vi "Enum Strings.vi"(11 "Enum":variant) -> (2 "Selected item":string, 3 "Strings":string[](array[string]), 5 "# items in Enum":i16)   [LabVIEW 2011, in "LV JSON.lvlib"]
uses:
  LV JSON.lvlib
panel:
  out "selected item":u32
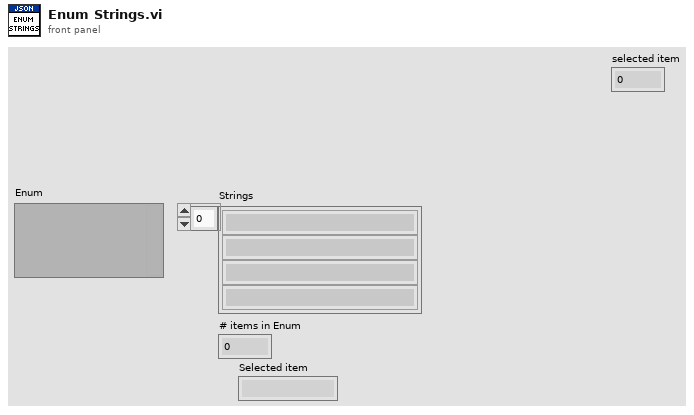
[diagram p1: front panel]
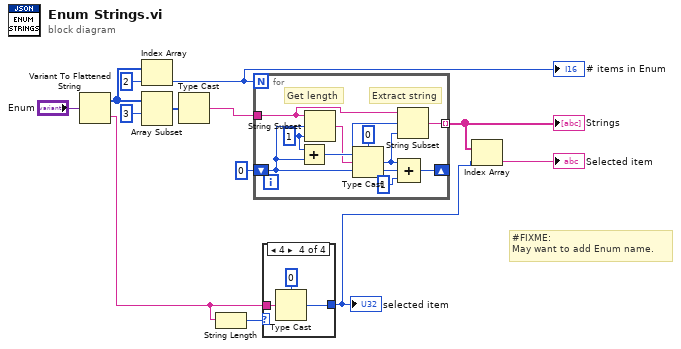
[diagram p0: block diagram]
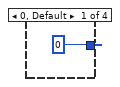
[diagram p2: hidden frame]
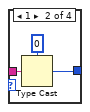
[diagram p3: hidden frame]
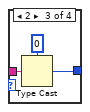
[diagram p4: hidden frame]
diagram:
  # "#FIXME:\nMay want to add Enum name."
  n1 = Variant To Flattened String(Variant="Enum") -> (data string=w4:string, 1:w11:i16[])
  n2 = Index Array(array=w11, index=2) -> (element=w9:i16)
  "# items in Enum" <- w9
  n3 = Array Subset(array=w11, index=3) -> (w13:i16[])  [unwired: 1 in]
  n4 = Type Cast(x=w13) -> (*(type *) &x=w7:string)  [unwired: 1 in]
  n5 = String Length(string=w4) -> (length=w5:i32)
  n6 = for {
    N: w9 -> [_]
    shift-right: [w23] -> _
    shift-left: 0 -> [w21]
    tunnel: w7 -> [w15]
    tunnel: [w17] -> w3 mode=indexing
    w20 = 1 ("length (rest)")
    # "Extract string"
    # "Get length"
    n7 = Add(x=w20, y=w21) -> (x+y=w19:i32)
    n8 = String Subset(string=w15, offset (0)=w21, length (rest)=w20) -> (substring=w16:string)
    n9 = Type Cast(type=u8 0, x=w16) -> (*(type *) &x=w18:u8)
    n10 = String Subset(string=w15, offset (0)=w19, length (rest)=w18) -> (substring=w17:string)
    n11 = Compound Arithmetic op=ADD(w18, w21, 1 ("length (rest)")) -> (w23:i32)
  }
  "Strings" <- w3
  n12 = case shown="4" w5 {
    tunnel: [u32 0 w25 w28 w31] -> w1
    tunnel: w4 -> [_ w27 w30 w33]
    frame 0, Default {
    }
    frame 1 {
      n13 = Type Cast(type=u8 0, x=w27) -> (*(type *) &x=w25:u8)
    }
    frame 2 {
      n14 = Type Cast(type=u16 0, x=w30) -> (*(type *) &x=w28:u16)
    }
    frame 4 {
      n15 = Type Cast(type=u32 0, x=w33) -> (*(type *) &x=w31:u32)
    }
  }
  "selected item" <- w1
  n16 = Index Array(array=w3, index=w1) -> (element=→"Selected item":string)
